vi "Write Buffer Size.vi"(8 "error in (no error)":errorcluster, 10 "Buffer Size":u32, 11 "Node Ptr":T1 format="%.0x") -> (0 "error out":errorcluster, 3 "Node Ptr out":T1 format="%.0x")   [LabVIEW 2019, in "UDP-Custom-Device System Explorer.lvlib" / "Buffered Data Packet.lvlib"]
uses:
  Buffered Data Packet.lvlib
  <vilib>/NI VeriStand/Custom Device API/Custom Device Item Ref.ctl
  Shared/Constants.vi
  <vilib>/NI VeriStand/Custom Device API/Set Item Property (U32).vi
  <vilib>/NI VeriStand/Custom Device API/Custom Device API.lvlib
  Shared/UDP-Custom-Device Shared.lvlib
  UDP-Custom-Device System Explorer.lvlib
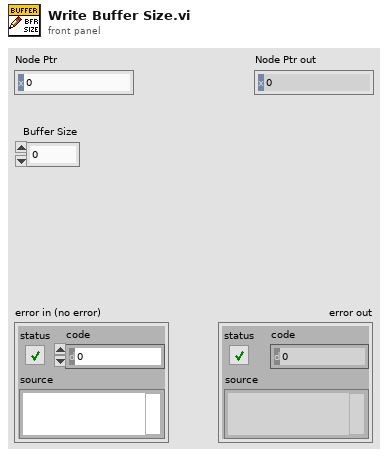
[diagram p1: front panel]
types:
  T1 = typedef "Custom Device API.lvlib/Custom Device Item Ref.ctl" = u64
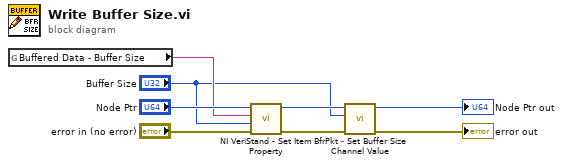
[diagram p0: block diagram]
diagram:
  n1 = global read "Constants.vi" "Buffered Data - Buffer Size"() -> (w6:string)
  n2 = call-poly <vilib>:"NI VeriStand - Set Item Property.vi"("error in (no error)"="error in (no error)", "Value"="Buffer Size", "Property Name"=w6, "Item Ref in"="Node Ptr") -> ("error out"=w3:errorcluster, "Item Ref out"=w5:T1)  [unwired: 5 in, 1 out]
  n3 = call "BfrPkt - Set Buffer Size Channel Value.vi"("error in (no error)"=w3, "Buffer Size"="Buffer Size", "Node Ptr"=w5) -> ("error out"=→"error out":errorcluster, "Node Ptr out"=→"Node Ptr out":T1)  [unwired: 7 in]
